vi "Apply PSRR Test.vi"(8 "error in (no error)":errorcluster, 11 "VISA resource name":refnum<visa-resource-name>) -> (0 "error out":errorcluster, 3 "VISA resource name out":refnum<visa-resource-name>)   [LabVIEW 2023, in "Keysight-DSQx3014T.lvlib"]
doc: "Applies the power supply rejection ratio (PSRR) analysis.\nUse Configure Power Analysis (Power Supply Rejection Ratio).vi to configure the PSRR analysis.\n\n<B>Note(s):</B>\n1) The Power Supply Rejection Ratio (PSRR) test is used to determine how well a voltage regulator rejects ripple noise over different frequency range.\n2) Do not use error query in this VI, because the instrument will not respond to any command during the PSRR test.\n3) This VI is only applicable for 6000 series."
uses:
  Keysight-DSQx3014T.lvlib
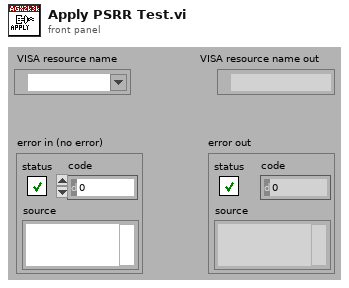
[diagram p1: front panel]
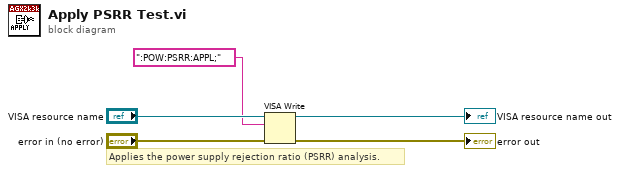
[diagram p0: block diagram]
diagram:
  # "Applies the power supply rejection ratio (PSRR) analysis."
  n1 = VISA Write(VISA resource name="VISA resource name", write buffer=":POW:PSRR:APPL;", error in (no error)="error in (no error)") -> (VISA resource name out=→"VISA resource name out":refnum<visa-resource-name>, error out=→"error out":errorcluster)  [unwired: 1 out]
